vi "AIT 1553 - Add Data Channel.vi"(8 "error in (no error)":errorcluster, 11 "Node Ptr":u64 format="%.0x") -> (0 "error out":errorcluster)   [LabVIEW 2013, in "AIT 1553 Custom Device.lvlib"]
uses:
  AIT 1553 Custom Device.lvlib
  <vilib>/NI Veristand/Custom Device API/Custom Device Channel.ctl
  <vilib>/NI Veristand/Custom Device API/Custom Device Channel Type.ctl
  Controls/1553 Param.ctl
  Controls and Global/Global.vi
  <vilib>/NI Veristand/Custom Device API/Get Item Property (U32).vi
  <vilib>/NI Veristand/Custom Device API/Get Item Property (U32 Array).vi
  <vilib>/NI Veristand/Custom Device API/Get Item Property (Boolean).vi
  <vilib>/NI Veristand/Custom Device API/Custom Device API.lvlib
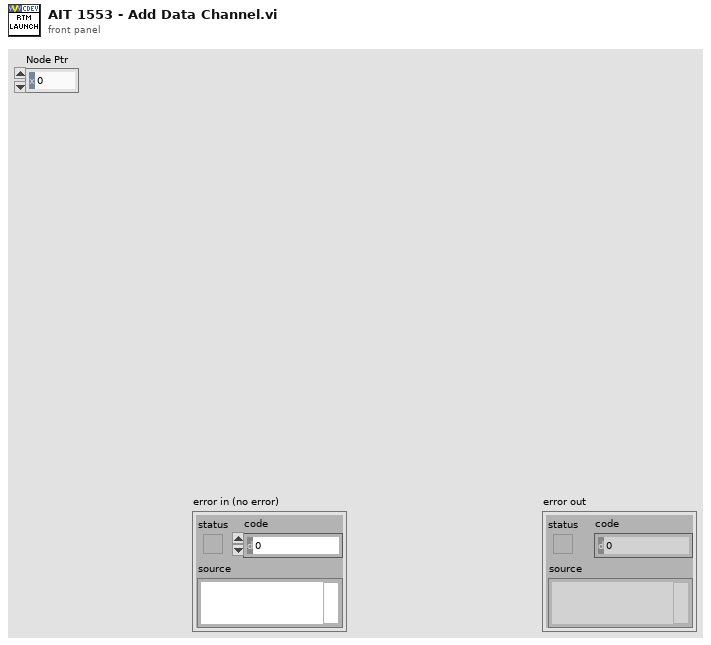
[diagram p1: front panel]
types:
  T1 = typedef "Custom Device API.lvlib/Custom Device Channel Type.ctl" = enum16{"Input", "Output"}
  T2 = typedef "AIT 1553 Custom Device.lvlib/1553 Param.ctl" = cluster{"name":string, "firstWord":i32, "startBit":i32, "numberBits":i32, "scaleFactor":dbl, "scaleOffset":dbl, "signed":bool}
  T3 = typedef "Custom Device API.lvlib/Custom Device Channel.ctl" = cluster{"Type":T1, "Units":string, "Default Value":dbl, "Faultable":bool, "Scalable":bool}
  T4 = typedef "Custom Device API.lvlib/Custom Device Item Ref.ctl" = u64
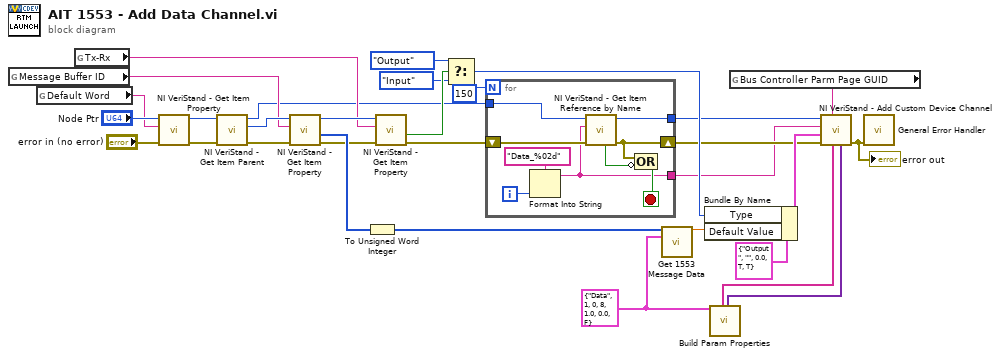
[diagram p0: block diagram]
diagram:
  w7 = T2 {"name"="Data", "firstWord"=1, "startBit"=0, "numberBits"=8, "scaleFactor"=1.0, "scaleOffset"=0.0, "signed"=FALSE} ("1553 Parameter")
  n1 = global read "Global.vi" "Message Buffer ID"() -> (w20:string)
  n2 = global read "Global.vi" "Default Word"() -> (w25:string)
  n3 = global read "Global.vi" "Tx-Rx"() -> (w14:string)
  n4 = call-poly <vilib>:"NI VeriStand - Get Item Property.vi"("error in (no error)"="error in (no error)", "Property Name"=w25, "Item Ref in"="Node Ptr") -> ("error out"=w27:errorcluster, "Item Ref out"=w28:T4)  [unwired: 5 in, 2 out]
  n5 = call <vilib>:"NI VeriStand - Get Item Parent.vi"("error in (no error)"=w27, "Item Ref in"=w28) -> ("error out"=w21:errorcluster, "Parent Ref"=w22:T4, "Item Ref out"=w4:T4)  [unwired: 6 in, 1 out]
  n6 = call-poly <vilib>:"NI VeriStand - Get Item Property.vi"("error in (no error)"=w21, "Property Name"=w20, "Item Ref in"=w22) -> ("error out"=w16:errorcluster, "Value"=w19:u32[], "Item Ref out"=w15:T4)  [unwired: 5 in, 1 out]
  n7 = To Unsigned Word Integer(number=w19) -> (unsigned 16bit integer=w18:u16[])
  n8 = call-poly <vilib>:"NI VeriStand - Get Item Property.vi"("error in (no error)"=w16, "Property Name"=w14, "Item Ref in"=w15) -> ("error out"=w6:errorcluster, "Value"=w13:bool)  [unwired: 5 in, 2 out]
  n9 = Select(t=Custom_Device_Channel_Type."Output" ("Type"), s=w13, f=Custom_Device_Channel_Type."Input" ("Type")) -> (s? t:f=w9:T1)
  n10 = for {
    N: 150 -> [_]
    tunnel: w4 -> [w40]
    tunnel: [w35] -> w3
    tunnel: [w32] -> w2
    shift-right: [w37] -> w5
    shift-left: w6 -> [w39]
    i -> [w34]
    stop <- w38 stop-if-true
    n11 = Format Into String(format string="Data_%02d" ("name"), w34) -> (resulting string=w32:string)  [unwired: 2 in, 1 out]
    n12 = call <vilib>:"NI VeriStand - Get Item Reference by Name.vi"("error in (no error)"=w39, "Item Name"=w32, "Parent Ref in"=w40) -> ("error out"=w37:errorcluster, "Parent Ref out"=w35:T4, "Found"=w36:bool)  [unwired: 5 in, 1 out]
    n13 = Compound Arithmetic op=OR(w37, invert w36) -> (w38:bool)
  }
  n14 = call "Get 1553 Message Data.vi"("MSG DATA"=w18, "1553 Parameter"=w7) -> ("Value"=w17:dbl)  [unwired: 12 in, 1 out]
  n15 = Bundle By Name(cluster=T3 {"Type"=enum."Output", "Units"="", "Default Value"=0.0, "Faultable"=TRUE, "Scalable"=TRUE} ("Channel"), "Type"=w9, "Default Value"=w17) -> (w8:T3)
  n16 = call "Build Param Properties.vi"("1553 Parameter"=w7) -> ("Prop Names"=w24:string[], "Prop Values"=w23:variant[])  [unwired: 10 in, 7 out]
  n17 = global read "Global.vi" "Bus Controller Parm Page GUID"() -> (w31:string)
  n18 = call <vilib>:"NI VeriStand - Add Custom Device Channel.vi"("Property Values"=w23, "Property names"=w24, "GUID (Default Channel)"=w31, "error in (no error)"=w5, "Channel"=w8, "Channel Name"=w2, "Parent Ref in"=w3) -> ("error out"=w30:errorcluster)  [unwired: 1 in, 3 out]
  "error out" <- w30
  n19 = call <vilib>:"General Error Handler.vi"("error in (no error)"=w30) -> ()  [unwired: 10 in, 5 out]
